vi "ScaleWayPoints.vi"(11 "WayPointCluster":T2) -> (0 "FPGA Way Points":i16[](array[numeric]), 2 "VelScallerCluster":T1, 3 ".not. x?":bool)   [LabVIEW 2023]
uses:
  TypeDefs/WayPointCluster.ctl
  TypeDefs/VelScallerCluster.ctl
  User_Vi/Settings.vi
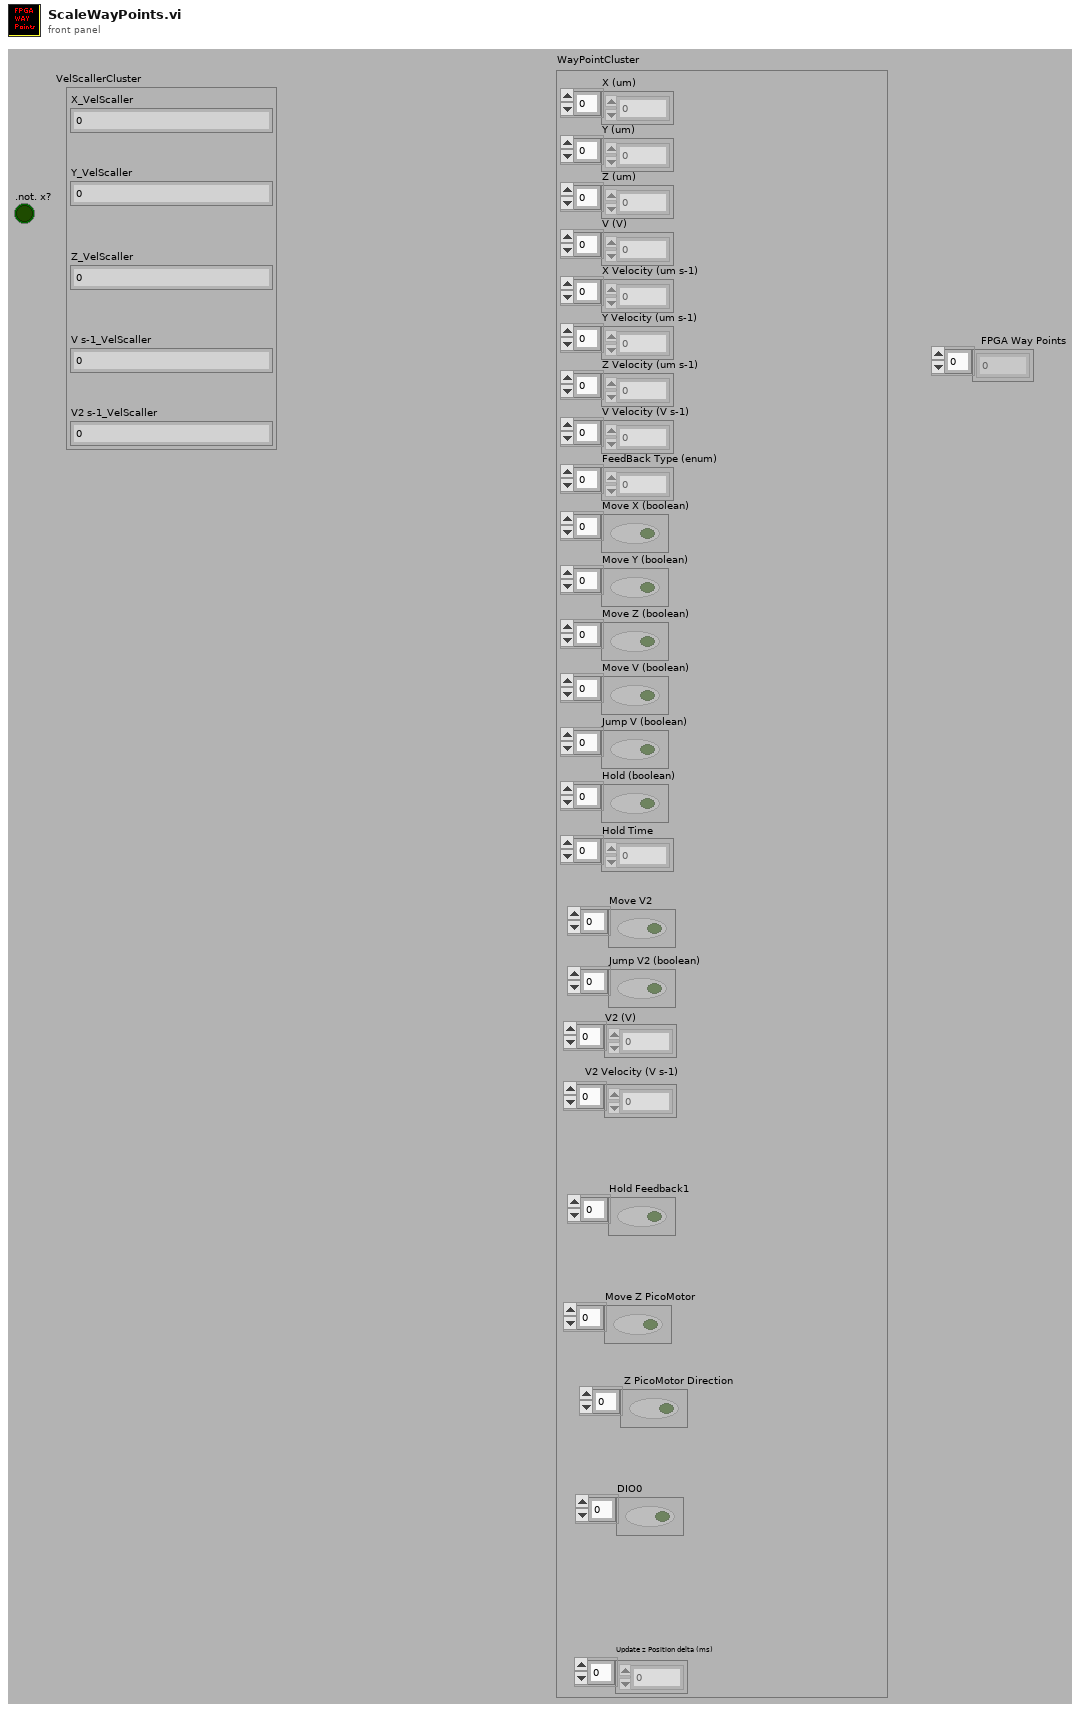
[diagram p1: front panel]
types:
  T1 = typedef "VelScallerCluster.ctl" = cluster{"X_VelScaller":i32, "Y_VelScaller":i32, "Z_VelScaller":i32, "V s-1_VelScaller":i32, "V2 s-1_VelScaller":i32}
  T2 = typedef "WayPointCluster.ctl" = cluster{"X (um)":dbl[], "Y (um)":dbl[], "Z (um)":dbl[], "V (V)":dbl[], "X Velocity (um s-1)":dbl[], "Y Velocity (um s-1)":dbl[], "Z Velocity (um s-1)":dbl[], "V Velocity (V s-1)":dbl[], "FeedBack Type (enum)":u16[], "Move X (boolean)":bool[], "Move Y (boolean)":bool[], "Move Z (boolean)":bool[], "Move V (boolean)":bool[], "Jump V (boolean)":bool[], "Hold (boolean)":bool[], "Hold Time":u32[], "V2 (V)":dbl[], "Move V2":bool[], "V2 Velocity (V s-1)":dbl[], "Jump V2 (boolean)":bool[], "Update z Position delta (ms)":i16[], "Hold Feedback1":bool[], "Move Z PicoMotor":bool[], " Z PicoMotor Direction":bool[], "DIO0":bool[]}
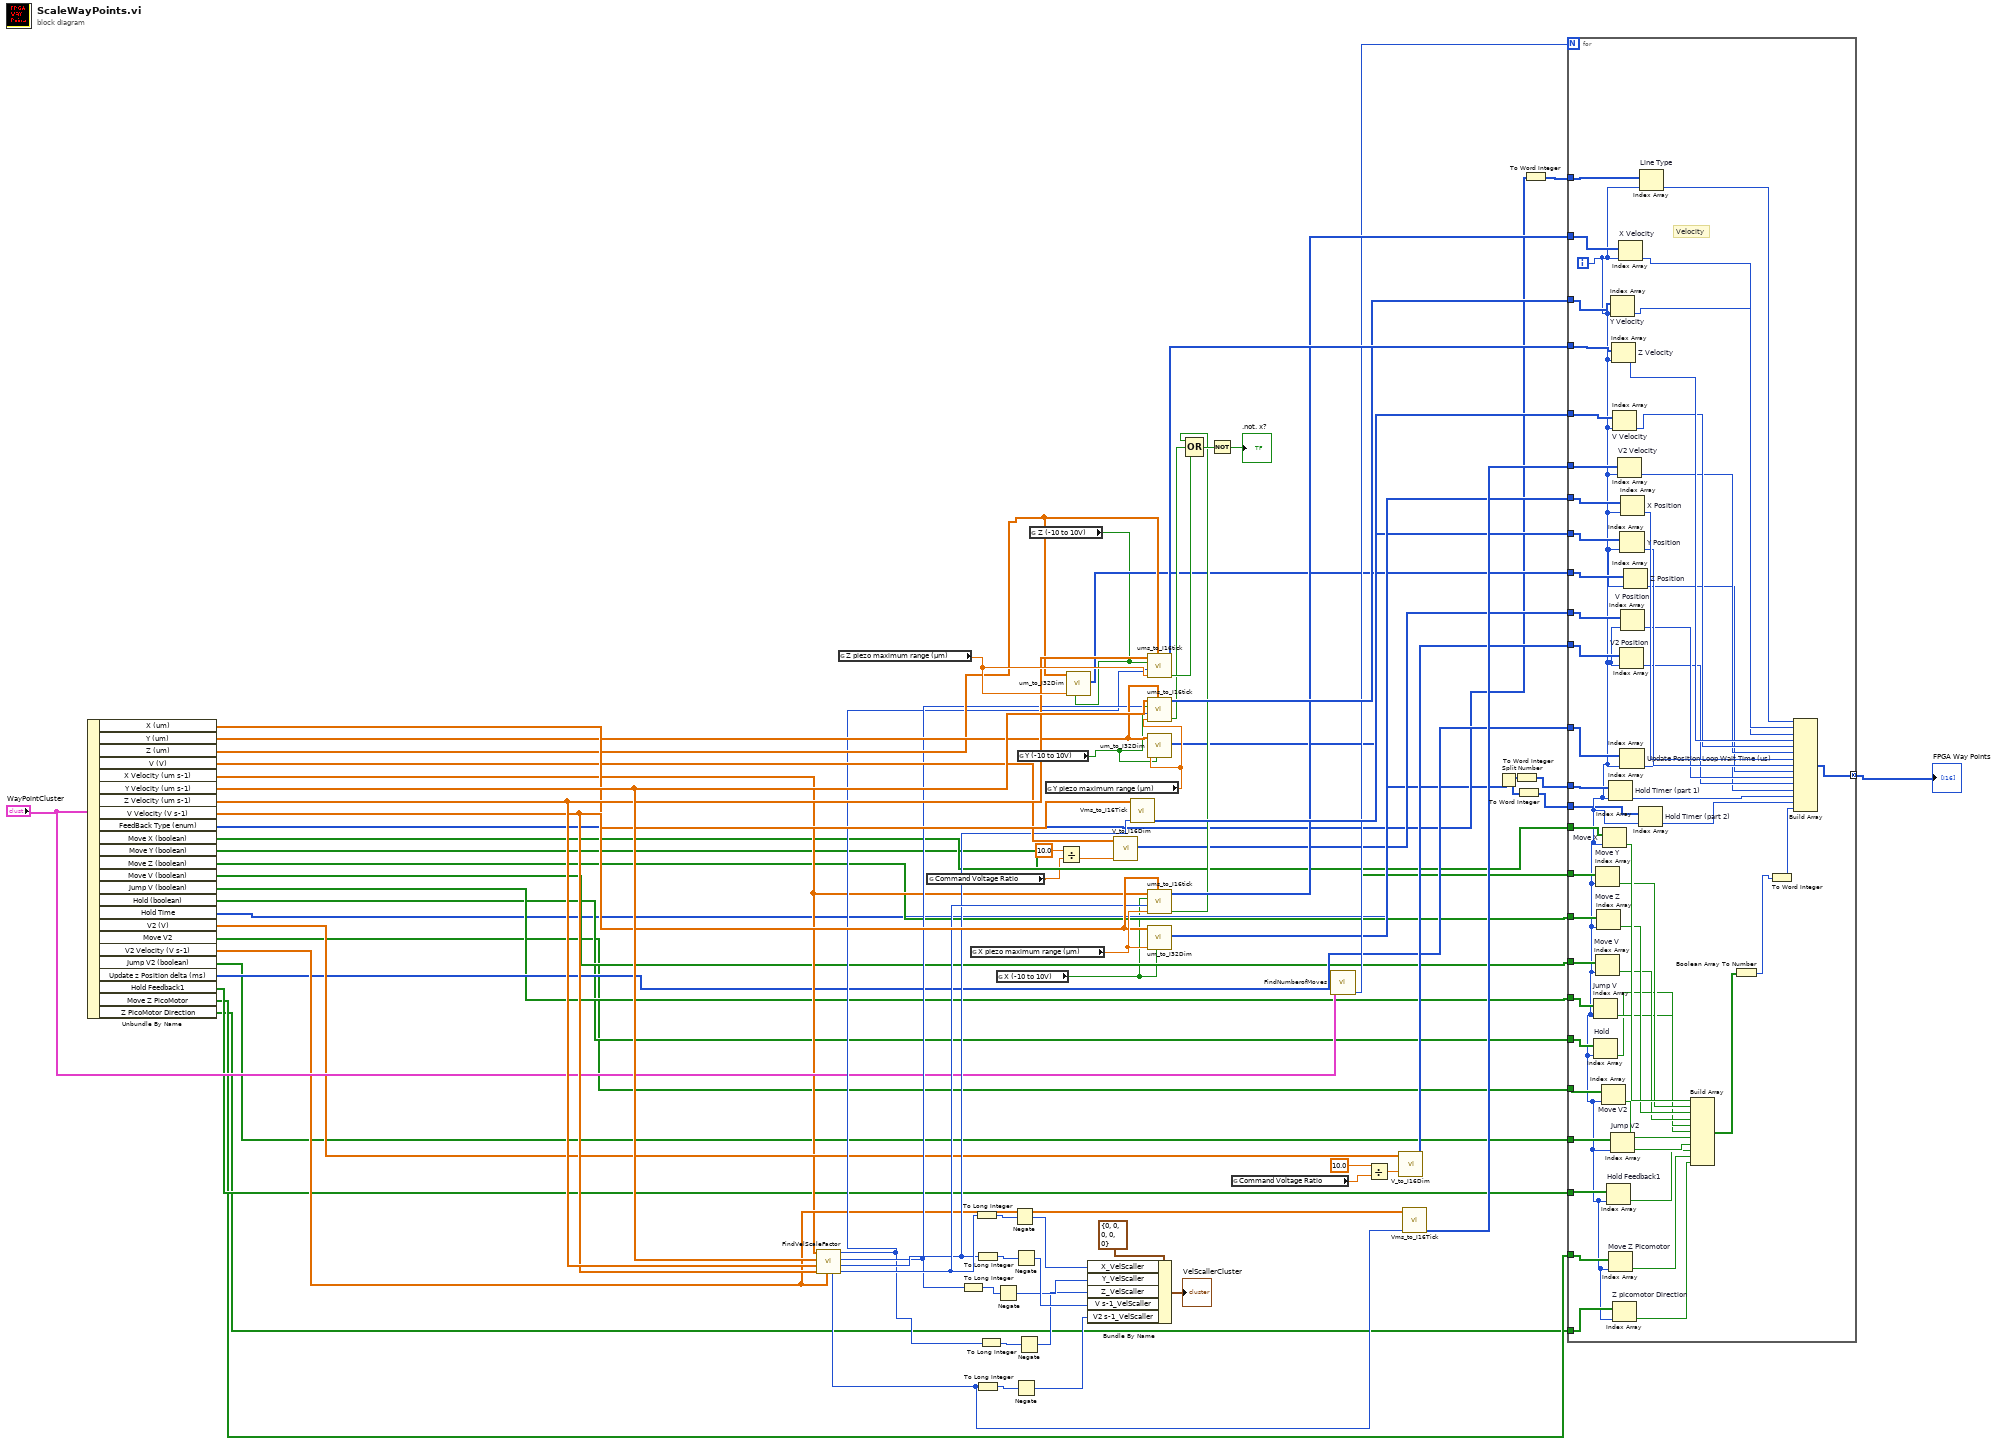
[diagram p0: block diagram]
diagram:
  n1 = Unbundle By Name("WayPointCluster") -> ("X (um)"=w60:dbl[], "Y (um)"=w59:dbl[], "Z (um)"=w58:dbl[], "V (V)"=w57:dbl[], "X Velocity (um s-1)"=w44:dbl[], "Y Velocity (um s-1)"=w64:dbl[], "Z Velocity (um s-1)"=w63:dbl[], "V Velocity (V s-1)"=w62:dbl[], "FeedBack Type (enum)"=w16:u16[], "Move X (boolean)"=w26:bool[], "Move Y (boolean)"=w25:bool[], "Move Z (boolean)"=w24:bool[], "Move V (boolean)"=w23:bool[], "Jump V (boolean)"=w22:bool[], "Hold (boolean)"=w21:bool[], "Hold Time"=w14:u32[], "V2 (V)"=w46:dbl[], "Move V2"=w20:bool[], "V2 Velocity (V s-1)"=w45:dbl[], "Jump V2 (boolean)"=w19:bool[], "Update z Position delta (ms)"=w27:i16[], "Hold Feedback1"=w17:bool[], "Move Z PicoMotor"=w6:bool[], "Z PicoMotor Direction"=w5:bool[])
  n2 = call "FindVelScaleFactor.vi"("V2 Velocity [V s-1]"=w45, "V Velocity [V s-1]"=w62, "Z Velocity [um s-1]"=w63, "Y Velocity [um s-1]"=w64, "X Velocity [um s-1]"=w44) -> ("X_VelScaller"=w56:u32, "V s-1_VelScaller"=w52:u32, "Y_VelScaller"=w51:u32, "Z_VelScaller"=w50:u32, "V2 s-1_VelScaller"=w43:u32)  [unwired: 2 in]
  n3 = global read "Settings.vi" "Z piezo maximum range (µm)"() -> (w67:dbl)
  n4 = global read "Settings.vi" "Command Voltage Ratio"() -> (w13:dbl)
  n5 = To Long Integer(number=w51) -> (32bit integer=w54:i32)
  n6 = global read "Settings.vi" "X piezo maximum range (µm)"() -> (w65:dbl)
  n7 = To Long Integer(number=w56) -> (32bit integer=w61:i32)
  n8 = To Long Integer(number=w52) -> (32bit integer=w55:i32)
  n9 = To Long Integer(number=w43) -> (32bit integer=w47:i32)
  n10 = To Long Integer(number=w50) -> (32bit integer=w53:i32)
  n11 = global read "Settings.vi" "X (-10 to 10V)"() -> (w12:bool)
  n12 = Negate(x=w54) -> (-x=w38:i32)
  n13 = Negate(x=w61) -> (-x=w40:i32)
  n14 = Negate(x=w55) -> (-x=w39:i32)
  n15 = Negate(x=w47) -> (-x=w36:i32)
  n16 = global read "Settings.vi" "Y (-10 to 10V)"() -> (w11:bool)
  n17 = Negate(x=w53) -> (-x=w37:i32)
  n18 = global read "Settings.vi" "Z (-10 to 10V)"() -> (w10:bool)
  n19 = global read "Settings.vi" "Y piezo maximum range (µm)"() -> (w66:dbl)
  n20 = Divide(x=10.0 ("Max/Min Value [V]"), y=w13) -> (x/y=w42:dbl)
  n21 = call "um_to_I32Dim.vi"("-10 to 10V?"=w10, "Max Value [um]"=w67, "Input"=w58) -> ("Array"=w30:i16[])  [unwired: 8 in]
  n22 = Bundle By Name(cluster=T1 {"X_VelScaller"=0, "Y_VelScaller"=0, "Z_VelScaller"=0, "V s-1_VelScaller"=0, "V2 s-1_VelScaller"=0} ("VelScallerCluster"), "X_VelScaller"=w40, "Y_VelScaller"=w38, "Z_VelScaller"=w37, "V s-1_VelScaller"=w39, "V2 s-1_VelScaller"=w36) -> (→"VelScallerCluster":T1)
  n23 = call "V_to_I16Dim.vi"("Max/Min Value [V]"=w42, "Input"=w57) -> ("16bit integer"=w29:i16[])  [unwired: 9 in]
  n24 = call "Vms_to_I16Tick.vi"("n"=w52, "V Velocity [V s-1]"=w62) -> ("V Velocity"=w76:i16[])  [unwired: 9 in]
  n25 = call "ums_to_I16tick.vi"("Positions"=w58, "Max piezo distance"=w67, "n"=w50, "-10 to +10V?"=w10, "Input Velocity"=w63) -> ("Error"=w70:bool, "Scalled Velocity"=w75:i16[])  [unwired: 3 in]
  n26 = call "ums_to_I16tick.vi"("Positions"=w59, "Max piezo distance"=w66, "n"=w51, "-10 to +10V?"=w11, "Input Velocity"=w64) -> ("Error"=w69:bool, "Scalled Velocity"=w74:i16[])  [unwired: 3 in]
  n27 = call "um_to_I32Dim.vi"("-10 to 10V?"=w11, "Max Value [um]"=w66, "Input"=w59) -> ("Array"=w31:i16[])  [unwired: 8 in]
  n28 = call "ums_to_I16tick.vi"("Positions"=w60, "Max piezo distance"=w65, "n"=w56, "-10 to +10V?"=w12, "Input Velocity"=w44) -> ("Error"=w68:bool, "Scalled Velocity"=w73:i16[])  [unwired: 3 in]
  n29 = call "um_to_I32Dim.vi"("-10 to 10V?"=w12, "Max Value [um]"=w65, "Input"=w60) -> ("Array"=w32:i16[])  [unwired: 8 in]
  n30 = Compound Arithmetic op=OR(w68, w69, w70) -> (w71:bool)
  n31 = Not(x=w71) -> (.not. x?=→".not. x?":bool)
  n32 = global read "Settings.vi" "Command Voltage Ratio"() -> (w9:dbl)
  n33 = call "FindNumberofMoves.vi"("WayPointCluster"="WayPointCluster") -> ("max length"=w48:i32)  [unwired: 10 in]
  n34 = Divide(x=10.0 ("Max/Min Value [V]"), y=w9) -> (x/y=w7:dbl)
  n35 = call "V_to_I16Dim.vi"("Max/Min Value [V]"=w7, "Input"=w46) -> ("16bit integer"=w28:i16[])  [unwired: 9 in]
  n36 = call "Vms_to_I16Tick.vi"("n"=w43, "V Velocity [V s-1]"=w45) -> ("V Velocity"=w33:i16[])  [unwired: 9 in]
  n37 = Split Number(x=w14) -> (hi(x)=w4:u16[], lo(x)=w2:u16[])
  n38 = To Word Integer(number=w4) -> (16bit integer=w3:i16[])
  n39 = To Word Integer(number=w2) -> (16bit integer=w1:i16[])
  n40 = To Word Integer(number=w16) -> (16bit integer=w15:i16[])
  n41 = for {
    N: w48 -> [_]
    tunnel: w76 -> [w128]
    tunnel: w75 -> [w129]
    tunnel: w74 -> [w130]
    tunnel: w73 -> [w131]
    tunnel: [w126] -> w18 mode=concatenating
    tunnel: w33 -> [w122]
    tunnel: w32 -> [w120]
    tunnel: w31 -> [w118]
    tunnel: w30 -> [w116]
    tunnel: w29 -> [w114]
    tunnel: w28 -> [w112]
    tunnel: w15 -> [w110]
    tunnel: w27 -> [w109]
    tunnel: w3 -> [w107]
    tunnel: w26 -> [w104]
    tunnel: w25 -> [w102]
    tunnel: w24 -> [w100]
    tunnel: w23 -> [w98]
    tunnel: w22 -> [w96]
    tunnel: w21 -> [w94]
    tunnel: w20 -> [w92]
    tunnel: w19 -> [w90]
    tunnel: w17 -> [w88]
    tunnel: w6 -> [w83]
    tunnel: w5 -> [w82]
    tunnel: w1 -> [w77]
    i -> [w79]
    # "Velocity"
    n42 = Index Array "Jump V"(array=w96, index=w79) -> (element=w95:bool)
    n43 = Index Array "Hold"(array=w94, index=w79) -> (element=w93:bool)
    n44 = Index Array "Move V"(array=w98, index=w79) -> (element=w97:bool)
    n45 = Index Array "Move Y"(array=w102, index=w79) -> (element=w101:bool)
    n46 = Index Array "Move Z"(array=w100, index=w79) -> (element=w99:bool)
    n47 = Index Array "Move V2"(array=w92, index=w79) -> (element=w91:bool)
    n48 = Index Array "Move X"(array=w104, index=w79) -> (element=w103:bool)
    n49 = Index Array "Hold Feedback1"(array=w88, index=w79) -> (element=w87:bool)
    n50 = Index Array "Hold Timer (part 1)"(array=w107, index=w79) -> (element=w106:i16)
    n51 = Index Array "Move Z Picomotor"(array=w83, index=w79) -> (element=w81:bool)
    n52 = Index Array "Y Velocity"(array=w130, index=w79) -> (element=w125:i16)
    n53 = Index Array "Jump V2"(array=w90, index=w79) -> (element=w89:bool)
    n54 = Index Array "Z Velocity"(array=w129, index=w79) -> (element=w124:i16)
    n55 = Index Array "V Velocity"(array=w128, index=w79) -> (element=w123:i16)
    n56 = Index Array "Z picomotor Direction"(array=w82, index=w79) -> (element=w80:bool)
    n57 = Index Array "V2 Velocity"(array=w122, index=w79) -> (element=w121:i16)
    n58 = Index Array "X Velocity"(array=w131, index=w79) -> (element=w127:i16)
    n59 = Index Array "V2 Position"(array=w112, index=w79) -> (element=w111:i16)
    n60 = Index Array "Y Position"(array=w118, index=w79) -> (element=w117:i16)
    n61 = Index Array "Update Position Loop Wait Time (us)"(array=w109, index=w79) -> (element=w108:i16)
    n62 = Index Array "X Position"(array=w120, index=w79) -> (element=w119:i16)
    n63 = Index Array "V Position"(array=w114, index=w79) -> (element=w113:i16)
    n64 = Index Array "Z Position"(array=w116, index=w79) -> (element=w115:i16)
    n65 = Index Array "Hold Timer (part 2)"(array=w77, index=w79) -> (element=w78:i16)
    n66 = Index Array "Line Type"(array=w110, index=w79) -> (element=w84:i16)
    n67 = Build Array(w103, w101, w99, w97, w95, w93, w91, w89, w87, w81, w80) -> (w105:bool[])
    n68 = Boolean Array To Number(Boolean array=w105) -> (number=w86:u16)
    n69 = To Word Integer(number=w86) -> (16bit integer=w85:i16)
    n70 = Build Array(w84, w127, w125, w124, w123, w121, w119, w117, w115, w113, w111, w108, w106, w78, w85) -> (w126:i16[])
  }
  "FPGA Way Points" <- w18
